vi "Wait_for_Button_Press_Trial.vi"() -> ()   [LabVIEW 2021]
panel:
  out "Numeric":i32
  in  "TAKE IMAGE":bool
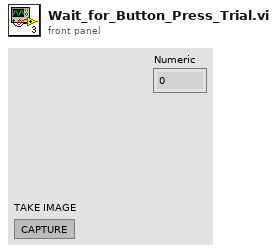
[diagram p1: front panel]
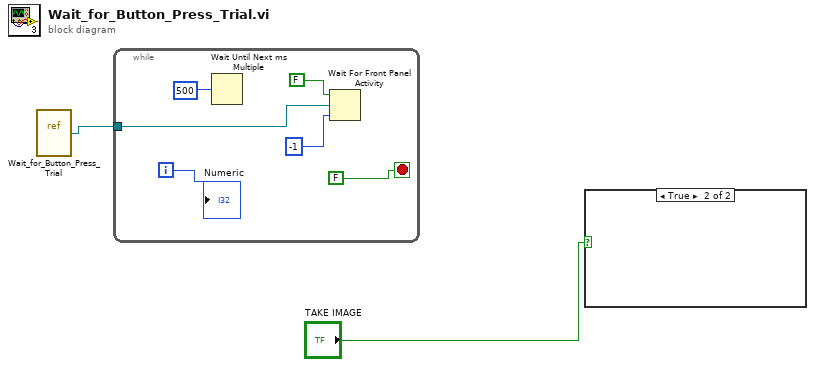
[diagram p0: block diagram]
diagram:
  n1 = vi-ref "Wait_for_Button_Press_Trial.vi"() -> (w2:refnum<vi>)
  n2 = while {
    tunnel: w2 -> [w4]
    i -> [w6]
    stop <- FALSE stop-if-true
    n3 = Wait Until Next ms Multiple(millisecond multiple=500) -> ()  [unwired: 1 out]
    n4 = Wait For Front Panel Activity(1:-1, 2:w4, 3:FALSE) -> ()  [unwired: 1 out]
    "Numeric" <- w6
  }
  n5 = case shown="True" "TAKE IMAGE" {
    frame False {
    }
    frame True {
    }
  }
